vi "1.4Modbus通讯实战.vi"() -> ()   [LabVIEW 2018]
uses:
  <vilib>/NI/Modbus Library/API/Wrapper/Create Serial Master.vi
  <vilib>/NI/Modbus Library/API/Master/Modbus Master.lvclass
  <vilib>/NI/Modbus Library/API/Wrapper/API Main.lvlib
panel:
  out "register values":u16[](array[numeric])
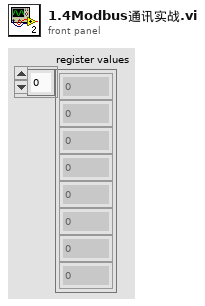
[diagram p1: front panel]
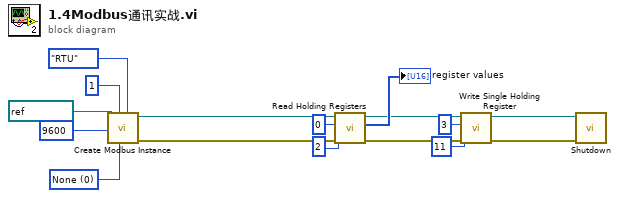
[diagram p0: block diagram]
diagram:
  w14 = u16 0 items=["None", "Odd", "Even", "Mark", "Space"] ("parity (even)")
  n1 = call-poly <vilib>:"Create Modbus Instance.vi"("serial type"=enum16{"RTU", "ASCII"}."RTU", "parity (even)"=w14, "unit ID"=u8 1, "baud rate"=u32 9600, "VISA resource name"=refnum<visa-resource-name> "COM2") -> ("error out"=w10:errorcluster, "serial master instance"=w11:refnum<class "Modbus Master.lvclass">)  [unwired: 5 in]
  n2 = call-dynamic "Read Holding Registers.vi"("error in"=w10, "number of inputs"=u16 2, "starting address"=u16 0, "Modbus master in"=w11) -> ("error out"=w4:errorcluster, "register values"=→"register values":u16[], "Modbus master out"=w6:refnum<class "Modbus Master.lvclass">)  [unwired: 5 in]
  n3 = call-dynamic "Write Single Holding Register.vi"("error in"=w4, "register to write"=u16 11, "address"=u16 3, "Modbus master in"=w6) -> ("error out"=w3:errorcluster, "Modbus master out"=w5:refnum<class "Modbus Master.lvclass">)  [unwired: 6 in]
  n4 = call-dynamic "Shutdown.vi"("error in"=w3, "Modbus master in"=w5) -> ()  [unwired: 9 in, 1 out]
